vi "decoding.vi"() -> ()   [LabVIEW 2019]
panel:
  out "Numeric":i32
  out "Array":u32[](array[numeric])
  in  "data out":string="\u0000\u0000æ\u001e\u0000\u0000\u0000\u0000\u0000\u0000\u0000\u0000\u0000\u0000\u0000\u0000\u0005\u0000[\u001d\u0001\u0000\u0013\u00002\u0001'\u0001\u0000%QT\u0001\u0000\u0001\u0000\u0001\u0000Uö\u0000\u00002\u0000\u0000\u0000\u0000\u0000\u0000\u0000"
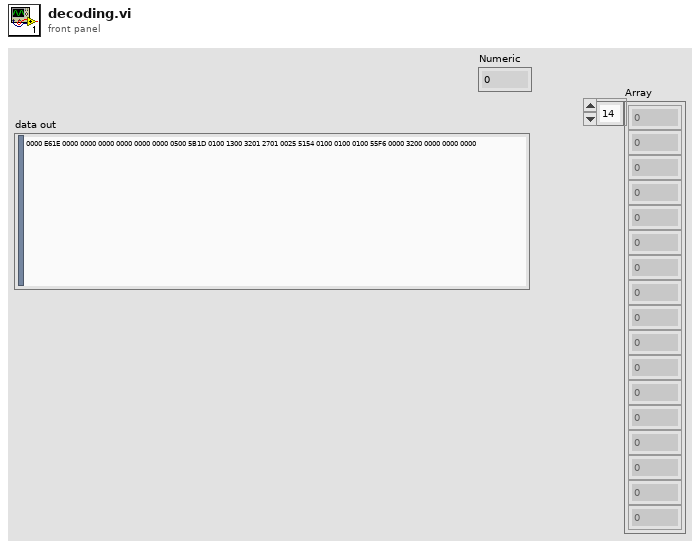
[diagram p1: front panel]
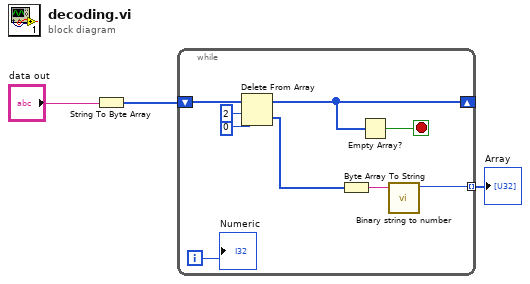
[diagram p0: block diagram]
diagram:
  n1 = String To Byte Array(string="data out") -> (unsigned byte array=w2:u8[])
  n2 = while {
    shift-right: [w10] -> _
    shift-left: w2 -> [w12]
    tunnel: [w7] -> w1 mode=indexing
    i -> [w6]
    stop <- w9 stop-if-true
    n3 = Delete From Array(array=w12, length=2, index=0) -> (deleted portion=w4:u8[], array with subset deleted=w10:u8[])
    n4 = Byte Array To String(unsigned byte array=w4) -> (string=w8:string)
    n5 = Empty Array?(array=w10) -> (empty?=w9:bool)
    n6 = call "Binary string to number.vi"("Binaty string"=w8) -> ("Numeric"=w7:u32)  [unwired: 10 in]
    "Numeric" <- w6
  }
  "Array" <- w1
